vi "AddElement.vi"(8 "error in":errorcluster, 9 "Name":string, 10 "OwningElement in":refnum<k20>, 11 "Document in":refnum<k20>) -> (0 "error out":errorcluster, 1 "NewElement":refnum<k20>, 2 "OwningElement out":refnum<k20>, 3 "Document out":refnum<k20>)   [LabVIEW 2021, in "ProligentXMLGenerator.lvlib" / "DOMSupport.lvlib"]
uses:
  DOMSupport.lvlib
  <resource>/objmgr/DOMUserDefRef.rc
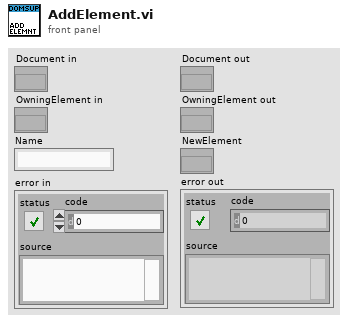
[diagram p1: front panel]
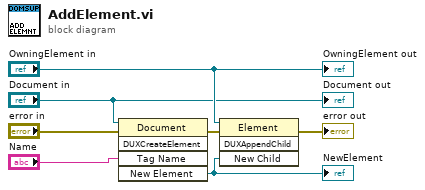
[diagram p0: block diagram]
diagram:
  n1 = invoke on="Invoke Node" class="Document" method="DUXCreateElement"(reference="Document in", error in="error in", "Tag Name"="Name") -> (error out=w6:errorcluster, "New Element"=w3:refnum<k20>)  [unwired: 2 in, 3 out]
  "NewElement" <- w3
  n2 = invoke on="Invoke Node" class="Element" method="DUXAppendChild"(reference="OwningElement in", error in=w6, "New Child"=w3) -> (error out=→"error out":errorcluster)  [unwired: 1 in, 3 out]
  "OwningElement out" <- "OwningElement in"
  "Document out" <- "Document in"
